vi "Configure.vi"(6 "GridSize":u32, 7 "Mode":u32, 8 "error in (no error)":errorcluster, 9 "Save":bool, 11 "AODAcq in":refnum<class "AODAcq.lvclass">) -> (0 "error out":errorcluster, 3 "AODAcq out":refnum<class "AODAcq.lvclass">)   [LabVIEW 2011, in "AODAcq.lvclass"]
uses:
  AODAcq.lvclass
  AODAcq.lvclass/AODAcq.ctl
  <vilib>/Utility/error.llb/Error Cluster From Error Code.vi
  Program Files/National Instruments/LabVIEW 2011/Targets/NI/FPGA/StockFPGA_IntfPrivate/ScriptTemplates/StockFPGA_PlugInRead32.vi
  <vilib>/rvi/errors/niLvFpgaAdjustHostInterfaceError.vi
  HDF5Tools/LabView/Create Dataset 2D Integer.vi
  <vilib>/rvi/interface/nirviReadWriteControl/nirviReadWriteControl.xnode
  FPGA_Control/AODRef.ctl
  FPGA Bitfiles/Acquisition_FPGATarget_AODControl(FPGA)_C1C38267.lvbitx
  FPGA_Control/AOD Control (FPGA).vi
  HDF5Tools/LabView/HDF5Tools.lvlib
  NiFpgaLv.dll
  <vilib>/FPGAPlugInAG/PXIe-7965R/niLvFpga_Read32_PXIe-7965R.vi
  <vilib>/rvi/interface/nirviReadWriteControl/niFpgaRWControlAccessTimeoutTemplate.vi
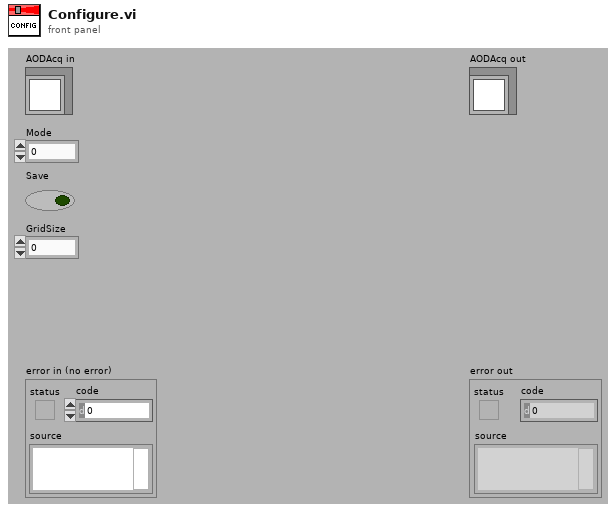
[diagram p1: front panel]
types:
  T1 = typedef "AODRef.ctl" = refnum<k20>
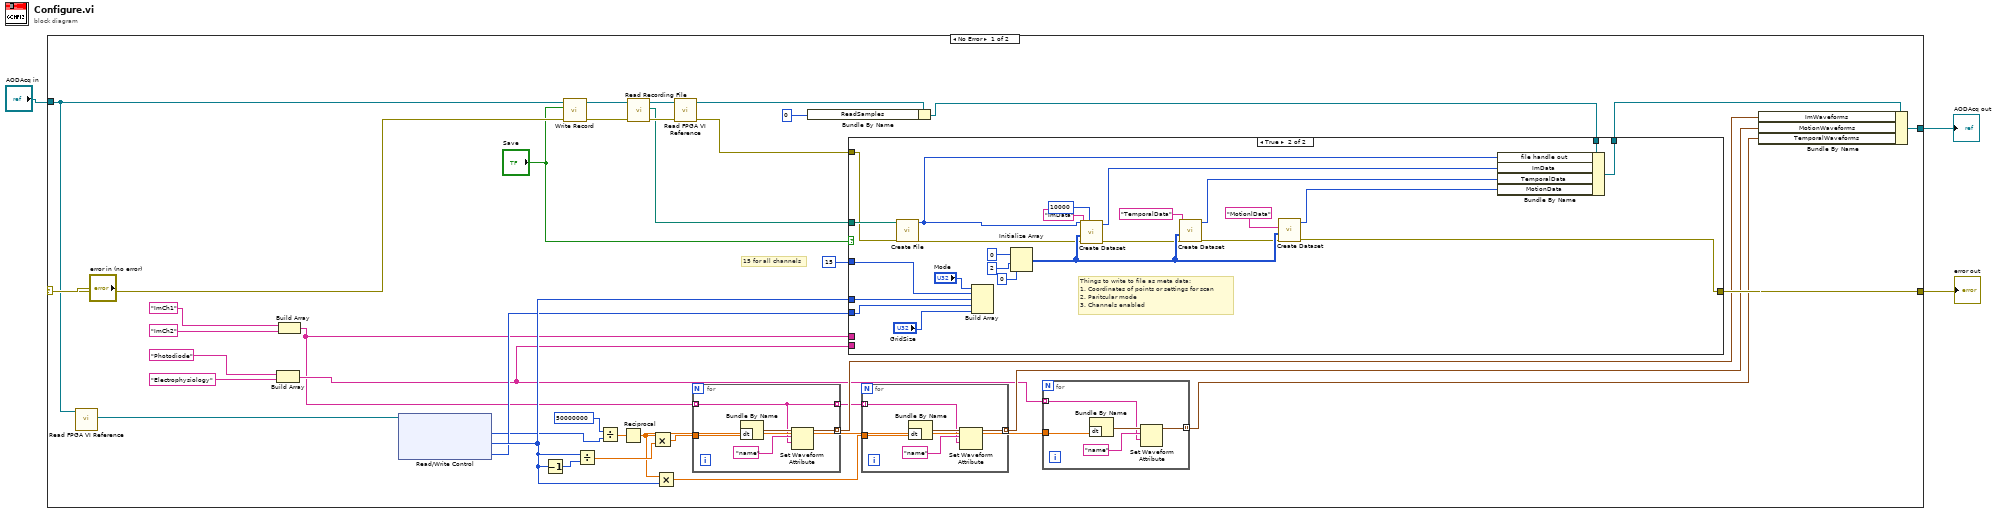
[diagram p0: block diagram]
diagram:
  n1 = case shown="No Error" "error in (no error)" {
    selector: "error in (no error)" -> [w11 w85]
    tunnel: [w41 w85] -> w3
    tunnel: [w31 w84] -> w1
    tunnel: "AODAcq in" -> [w12 w84]
    frame No Error {
      # "15 for all channels"
      n2 = call-dynamic "Read FPGA VI Reference.vi"("AODAcq in"=w12) -> ("FPGA VI Reference"=w34:T1)  [unwired: 8 in, 2 out]
      n3 = Build Array("Photodiode", "Electrophysiology") -> (w18:string[])
      n4 = Build Array("ImCh1", "ImCh2") -> (w17:string[])
      n5 = xnode "Read/Write Control"("FPGA VI Reference In"=w34) -> ("Setup.Downsample"=w13:u32, "Scan.Motion Increment"=w20:u32, "Scan.NumMotionPoints"=w19:u32)  [unwired: 1 in, 2 out]
      n6 = Decrement(x=w20) -> (x-1=w27:u32)
      n7 = call-dynamic "Write Record.vi"("error in (no error)"=w11, "Record"="Save", "AODAcq in"=w12) -> ("error out"=w7:errorcluster, "AODAcq out"=w9:refnum<class "AODAcq.lvclass">)  [unwired: 7 in]
      n8 = Divide(x=w20, y=w27) -> (x/y=w26:dbl)
      n9 = Divide(x=50000000, y=w13) -> (x/y=w36:dbl)
      n10 = Reciprocal(x=w36) -> (1/x=w25:dbl)
      n11 = call-dynamic "Read Recording File.vi"("error in (no error)"=w7, "AcquistionObject in"=w9) -> ("error out"=w6:errorcluster, "Recording File"=w5:path, "AcquistionObject out"=w8:refnum<class "AODAcq.lvclass">)  [unwired: 7 in]
      n12 = Multiply(x=w25, y=w26) -> (x*y=w28:dbl)
      n13 = Multiply(x=w25, y=w20) -> (x*y=w24:dbl)
      n14 = call-dynamic "Read FPGA VI Reference.vi"("error in (no error)"=w6, "AODAcq in"=w8) -> ("error out"=w29:errorcluster, "AODAcq out"=w30:refnum<class "AODAcq.lvclass">)  [unwired: 7 in, 1 out]
      n15 = for {
        tunnel: w17 -> [w52] mode=indexing
        tunnel: w28 -> [w56]
        tunnel: [w53] -> w33 mode=indexing
        tunnel: [w52] -> w23 mode=indexing
        n16 = Bundle By Name("dt"=w56) -> (w55:waveform(dbl))  [unwired: 1 in]
        n17 = Set Waveform Attribute(5:w52, 6:"name" ("name"), 7:w55) -> (3:w53:waveform(dbl))  [unwired: 1 in, 2 out]
      }
      n18 = Bundle By Name(cluster=w30, "ReadSamples"=u64 0) -> (w39:refnum<class "AODAcq.lvclass">)
      n19 = case shown="True" "Save" {
        tunnel: w5 -> [_ w76]
        tunnel: w39 -> [w58 w82]
        tunnel: [w58 w81] -> w32
        tunnel: w29 -> [w57 w75]
        tunnel: [w57 w60] -> w41
        tunnel: w17 -> [_ _]
        tunnel: w18 -> [_ _]
        tunnel: w20 -> [_ w79]
        tunnel: w19 -> [_ w80]
        tunnel: u32 15 -> [_ w78]
        frame False {
        }
        frame True {
          # "Things to write to file as meta data:\n1. Coordinates of points or settings for scan\n2. Paritcular mode\n3. Channels enabled"
          n20 = call "Create File.vi"("Error in"=w75, "File Name"=w76) -> ("Error out"=w66:errorcluster, "file_id"=w67:i32)  [unwired: 6 in]
          n21 = Build Array("Mode", w78, w79, w80, "GridSize") -> ()  [unwired: 1 out]
          n22 = Initialize Array(0, 2 ("dimension size"), 0 ("dimension size")) -> (w72:i32[][])
          n23 = call-poly "Create Dataset.vi"("Chunk size"=10000, "error in (no error)"=w66, "Datatype"=w72, "Dataset name"="ImData", "Location id in"=w67) -> ("error out"=w65:errorcluster, "Dataset id"=w63:i32)  [unwired: 5 in]
          n24 = call-poly "Create Dataset.vi"("error in (no error)"=w65, "Datatype"=w72, "Dataset name"="TemporalData") -> ("error out"=w64:errorcluster, "Dataset id"=w62:i32)  [unwired: 7 in]
          n25 = call-poly "Create Dataset.vi"("error in (no error)"=w64, "Datatype"=w72, "Dataset name"="MotionlData") -> ("error out"=w60:errorcluster, "Dataset id"=w61:i32)  [unwired: 7 in]
          n26 = Bundle By Name(cluster=w82, "file handle out"=w67, "ImData"=w63, "TemporalData"=w62, "MotionData"=w61) -> (w81:refnum<class "AODAcq.lvclass">)
        }
      }
      n27 = for {
        tunnel: w23 -> [w43] mode=indexing
        tunnel: w24 -> [w46]
        tunnel: [w42] -> w21 mode=indexing
        n28 = Bundle By Name("dt"=w46) -> (w45:waveform(dbl))  [unwired: 1 in]
        n29 = Set Waveform Attribute(5:w43, 6:"name" ("name"), 7:w45) -> (3:w42:waveform(dbl))  [unwired: 1 in, 2 out]
      }
      n30 = for {
        tunnel: w18 -> [w48] mode=indexing
        tunnel: w25 -> [w51]
        tunnel: [w47] -> w22 mode=indexing
        n31 = Bundle By Name("dt"=w51) -> (w50:waveform(dbl))  [unwired: 1 in]
        n32 = Set Waveform Attribute(5:w48, 6:"name" ("name"), 7:w50) -> (3:w47:waveform(dbl))  [unwired: 1 in, 2 out]
      }
      n33 = Bundle By Name(cluster=w32, "ImWaveforms"=w33, "MotionWaveforms"=w21, "TemporalWaveforms"=w22) -> (w31:refnum<class "AODAcq.lvclass">)
    }
    frame Error {
    }
  }
  "error out" <- w3
  "AODAcq out" <- w1
